vi "TDMS In Memory Write and Read.vi"() -> ()   [LabVIEW 2023]
doc: "This example demonstrates how to write data to a .tdms file in memory and read data from that file using the TDMS In Memory functions."
panel:
  out "File Size (byte)":i64
  out "Waveform Graph":i32[](graph)
  # "Overview: Demonstrates the use of the TDMS In Memory functions to write data to a .tdms file in memory and read data from that file.\nInstructions:\n1. Run this VI. Waveform Graph displays the data read from the .tdms file in memory. File Size (byte) returns the size of the .tdms file in memory.\n2. Delete the TDMS file (located at  [LabVIEW Data]\\Example TDMS In Memory Write and Read.tdms) when you are done."
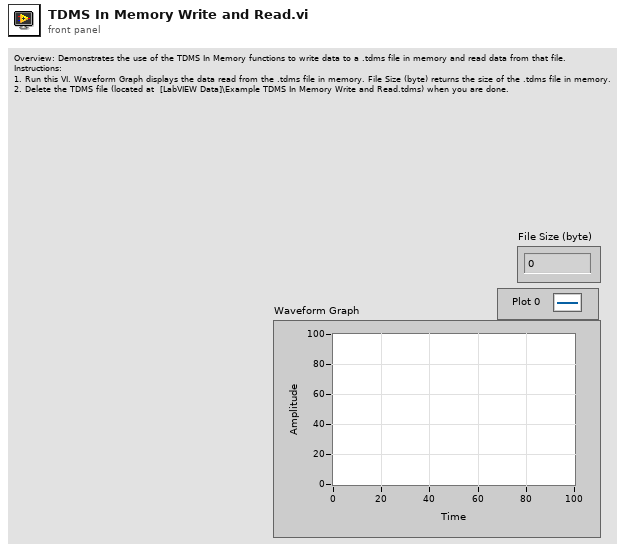
[diagram p1: front panel]
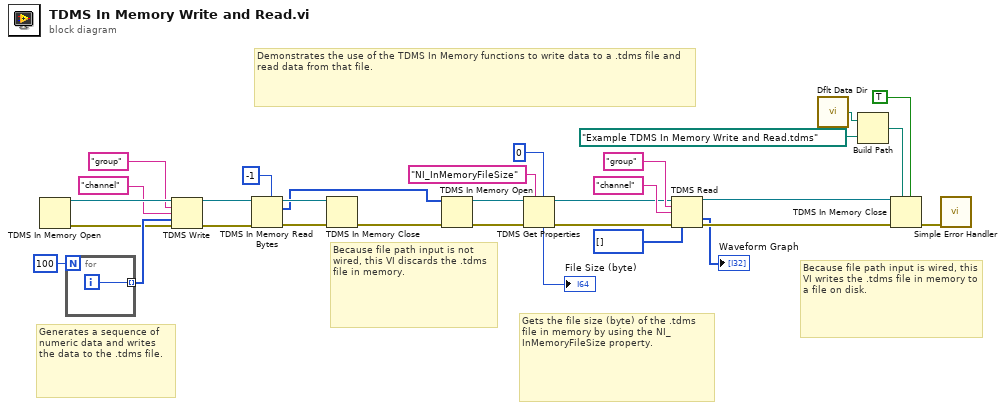
[diagram p0: block diagram]
diagram:
  # "Gets the file size (byte) of the .tdms file in memory by using the NI_InMemoryFileSize property."
  # "Generates a sequence of numeric data and writes the data to the .tdms file."
  # "Demonstrates the use of the TDMS In Memory functions to write data to a .tdms file and read data from that file."
  # "Because file path input is wired, this VI writes the .tdms file in memory to a file on disk."
  # "Because file path input is not wired, this VI discards the .tdms file in memory."
  n1 = TDMS In Memory Open() -> (0:w26:errorcluster, 3:w29:refnum<k34>)  [unwired: 2 in]
  n2 = for {
    N: 100 -> [_]
    tunnel: [w32] -> w27 mode=indexing
    i -> [w32]
  }
  n3 = TDMS Write(0:w29, 5:"group" ("group name in (Untitled)"), 7:"channel", 9:w27, 11:w26) -> (4:w24:refnum<k34>, 15:w8:errorcluster)  [unwired: 1 in, 2 out]
  n4 = TDMS In Memory Read Bytes(5:i64 -1 ("byte count (-1: all)"), 8:w8, 11:w24) -> (0:w7:errorcluster, 2:w5:u8[], 3:w9:refnum<k34>)  [unwired: 1 in]
  n5 = TDMS In Memory Close(8:w7, 11:w9) -> (0:w4:errorcluster)  [unwired: 2 in]
  n6 = TDMS In Memory Open(8:w4, 11:w5) -> (0:w15:errorcluster, 3:w16:refnum<k34>)
  n7 = TDMS Get Properties(5:i64 0, 7:"NI_InMemoryFileSize" ("property name"), 8:w15, 11:w16) -> (0:w13:errorcluster, 3:w14:refnum<k34>, 4:→"File Size (byte)":i64)  [unwired: 2 in, 3 out]
  n8 = TDMS Read(0:w14, 5:"group" ("group name in"), 7:"channel", 11:w13, 12:i32[] []) -> (4:w23:refnum<k34>, 10:→"Waveform Graph":i32[], 15:w22:errorcluster)  [unwired: 3 in, 3 out]
  n9 = call <vilib>:"Dflt Data Dir.vi"() -> ("App:Default Data Directory"=w31:path)
  n10 = Build Path(base path=w31, name or relative path=path "Example TDMS In Memory Write and Read.tdms") -> (appended path=w2:path)
  n11 = TDMS In Memory Close(5:TRUE ("overwrite (F)"), 7:w2, 8:w22, 11:w23) -> (0:w3:errorcluster)
  n12 = call <vilib>:"Simple Error Handler.vi"("error in (no error)"=w3) -> ()  [unwired: 4 in, 5 out]
